vi "ReferencedVariables_DeleteReferenceVariable_4x4x4.vi"(8 "error in (no error)":errorcluster, 11 "reference in":refnum<class>) -> (0 "error out":errorcluster, 2 "VariableReference":T1, 3 "reference out":refnum<class>)   [LabVIEW 2020]
doc: "This VI deletes a DVR reference variable."
uses:
  ReferencedVariable.ctl
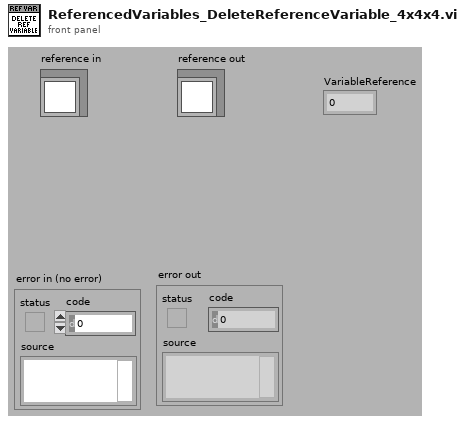
[diagram p1: front panel]
types:
  T1 = typedef "ReferencedVariable.ctl" = i32
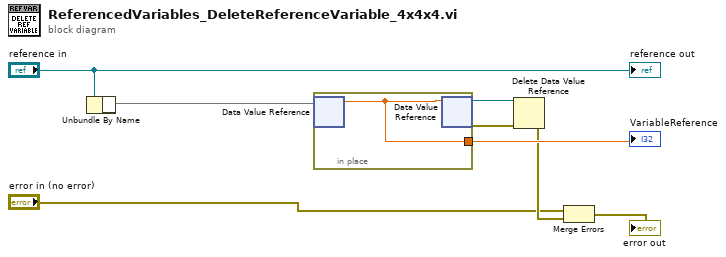
[diagram p0: block diagram]
diagram:
  n1 = Unbundle By Name("reference in") -> (w7)
  n2 = in-place {
    in-place-border: [w9] -> w6
    n3 = in-place-dvr #1(w7) -> (w9:dbl)  [unwired: 1 out]
    n4 = in-place-dvr #1(w9) -> (w5:refnum<data-value>, w4:errorcluster)
  }
  "VariableReference" <- w6
  n5 = Delete Data Value Reference(data value reference=w5, error in=w4) -> (error out=w3:errorcluster)  [unwired: 1 out]
  n6 = Merge Errors("error in (no error)", w3) -> (→"error out":errorcluster)
  "reference out" <- "reference in"
